vi "Experiment header-file operations.vi"(7 "Header file actions":T2, 8 "error in (no error)":errorcluster, 10 "Section Refs":T1[](array[typedef]), 11 "Path":path) -> (0 "error out":errorcluster)   [LabVIEW 2017]
uses:
  Typedefs/Header file actions.ctl
  Typedefs/Header file section refs.ctl
  <vilib>/Utility/config.llb/Config Data RefNum.ctl
  <vilib>/Utility/config.llb/NI_LVConfig.lvlib
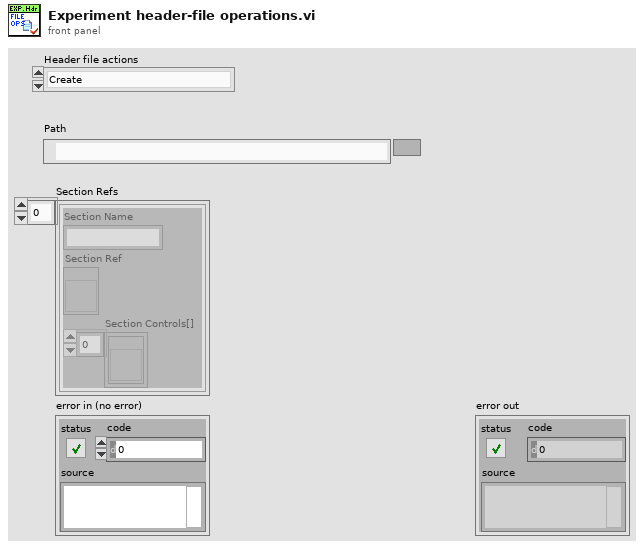
[diagram p1: front panel]
types:
  T1 = typedef "Header file section refs.ctl" = cluster{"Section Name":string, "Section Ref":refnum<vi>, "Section Controls[]":refnum<vi>[]}
  T2 = typedef "Header file actions.ctl" = enum16{"Create", "Open", "Read All", "Read Section", "Write All", "Write Section", "Close"}
  T3 = typedef "NI_LVConfig.lvlib/Config Data RefNum.ctl" = refnum<k1>
  T4 = typedef "Header file parameter names.ctl" = cluster{"Section Name":string, "Array":cluster{"Parameter name":string, "Control ref":refnum<vi>}[]}
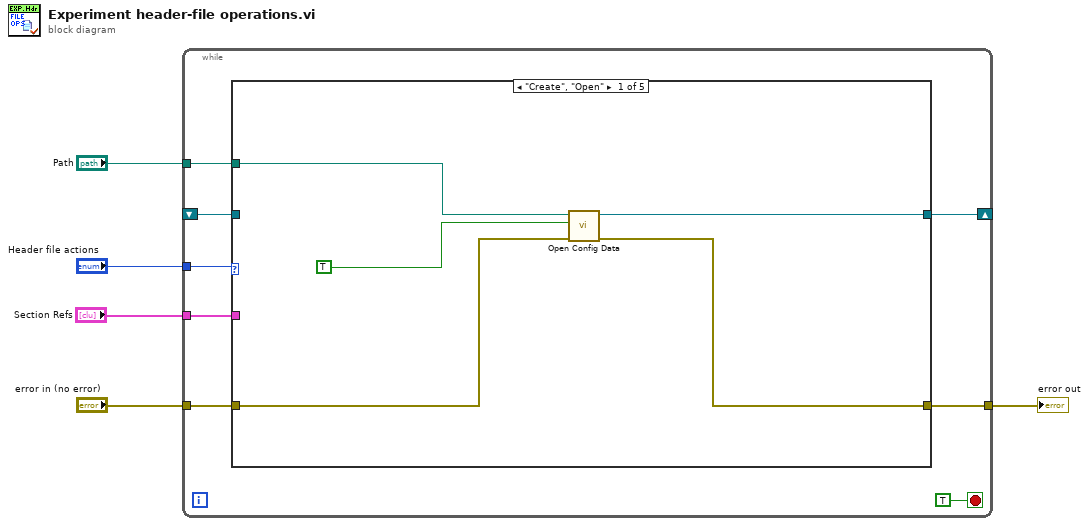
[diagram p0: block diagram]
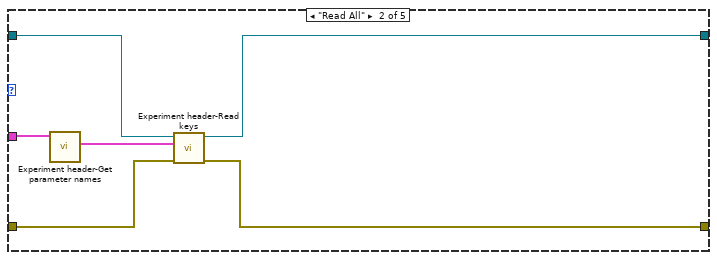
[diagram p2: hidden frame]
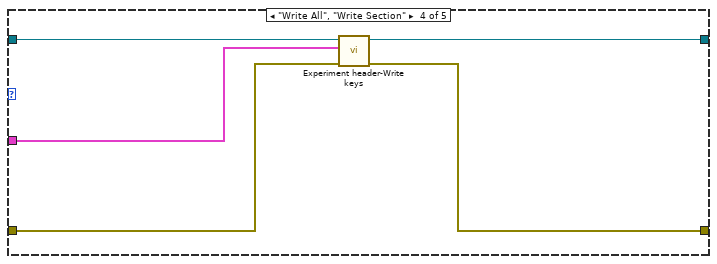
[diagram p4: hidden frame]
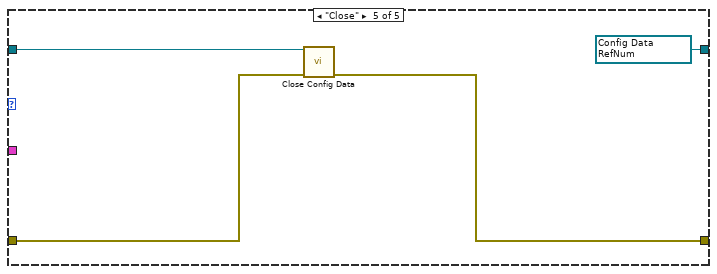
[diagram p5: hidden frame]
diagram:
  n1 = while {
    tunnel: "Header file actions" -> [w12]
    shift-right: [w11] -> _
    shift-left: _ -> [w7]
    tunnel: "Path" -> [w10]
    tunnel: "error in (no error)" -> [w9]
    tunnel: [w8] -> w2
    tunnel: "Section Refs" -> [w6]
    stop <- TRUE stop-if-true
    n2 = case shown="\"Create\", \"Open\"" w12 {
      tunnel: [w17 w19 w26 w30 w33] -> w11
      tunnel: w10 -> [w16 _ _ _ _]
      tunnel: w9 -> [w15 w23 w25 w28 w34]
      tunnel: [w14 w22 w25 w27 w32] -> w8
      tunnel: w7 -> [_ w20 w26 w31 w35]
      tunnel: w6 -> [_ w24 _ w29 _]
      frame "Create", "Open" {
        n3 = call <vilib>:"Open Config Data.vi"("error in (no error)"=w15, "create file if necessary (T)"=TRUE, "configuration file path"=w16) -> ("error out"=w14:errorcluster, "refnum"=w17:T3)  [unwired: 6 in, 1 out]
      }
      frame "Read All" {
        n4 = call "Experiment header-Get parameter names.vi"("Section Refs"=w24) -> ("All Parameter names"=w21:T4[])  [unwired: 8 in, 2 out]
        n5 = call "Experiment header-Read keys.vi"("error in (no error)"=w23, "All Parameter names"=w21, "FIle refnum IN"=w20) -> ("error out"=w22:errorcluster, "FIle refnum OUT"=w19:T3)  [unwired: 7 in]
      }
      frame "Read Section" {
      }
      frame "Write All", "Write Section" {
        n6 = call "Experiment header-Write keys.vi"("error in (no error)"=w28, "Section Refs"=w29, "FIle refnum IN"=w31) -> ("error in (no error) 2"=w27:errorcluster, "FIle refnum OUT"=w30:T3)  [unwired: 7 in]
      }
      frame "Close" {
        w33 = T3 refnum items=["config data"] ("FIle refnum OUT")
        n7 = call <vilib>:"Close Config Data.vi"("error in (no error)"=w34, "refnum"=w35) -> ("error out"=w32:errorcluster)  [unwired: 8 in, 1 out]
      }
    }
  }
  "error out" <- w2
